vi "ParseStateMsg.vi"(0 "StateMsg":refnum<class "JSON Object.lvclass">, 11 "error in":errorcluster) -> (4 "StateMsg":T1, 15 "error out":errorcluster)   [LabVIEW 2017]
uses:
  <vilib>/NI/JSON Support for LabVIEW/JSON Data Classes/JSON Object/JSON Object.lvclass
  StateMsg.ctl
  <vilib>/NI/JSON Support for LabVIEW/JSON Data Classes/JSON Object/Get Value (Object).vi
  <vilib>/NI/JSON Support for LabVIEW/JSON Data Classes/JSON Object/Get Value (String Value).vi
  <vilib>/NI/JSON Support for LabVIEW/JSON Data Classes/JSON Object/Get Value (Boolean Value).vi
  <vilib>/NI/JSON Support for LabVIEW/JSON Data Classes/JSON Object/Get Value (Numeric Value).vi
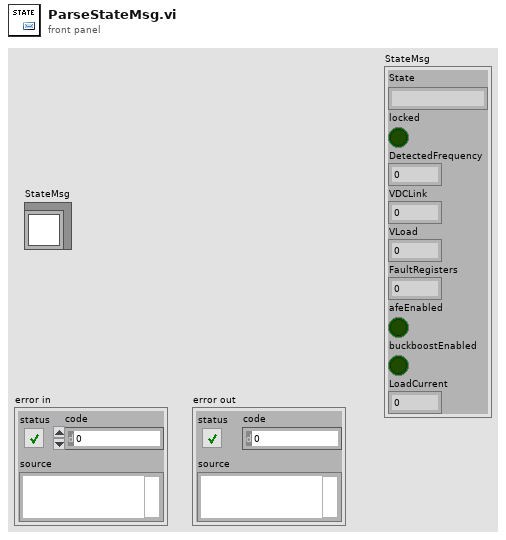
[diagram p1: front panel]
types:
  T1 = typedef "StateMsg.ctl" = cluster{"State":string, "locked":bool, "DetectedFrequency":dbl, "VDCLink":dbl, "VLoad":dbl, "FaultRegisters":u64, "afeEnabled":bool, "buckboostEnabled":bool, "LoadCurrent":dbl}
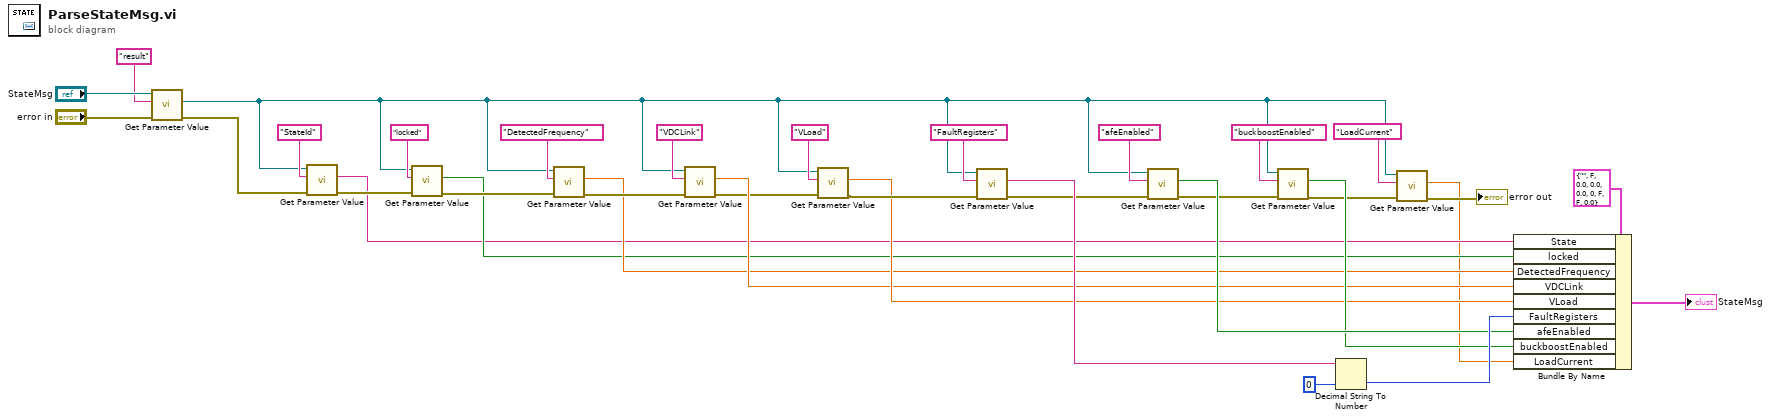
[diagram p0: block diagram]
diagram:
  n1 = call-poly <vilib>:"Get Parameter Value.vi"("error in (no error)"="error in", "key"="result", "JSON Object in"="StateMsg") -> ("error out"=w18:errorcluster, "value"=w5:refnum<class "JSON Object.lvclass">)  [unwired: 7 in]
  n2 = call-poly <vilib>:"Get Parameter Value.vi"("error in (no error)"=w18, "key"="StateId", "JSON Object in"=w5) -> ("error out"=w29:errorcluster, "value"=w6:string)  [unwired: 7 in]
  n3 = call-poly <vilib>:"Get Parameter Value.vi"("error in (no error)"=w29, "key"="locked", "JSON Object in"=w5) -> ("error out"=w28:errorcluster, "value"=w7:bool)  [unwired: 7 in]
  n4 = call-poly <vilib>:"Get Parameter Value.vi"("error in (no error)"=w28, "key"="DetectedFrequency", "JSON Object in"=w5) -> ("error out"=w27:errorcluster, "value"=w8:dbl)  [unwired: 7 in]
  n5 = call-poly <vilib>:"Get Parameter Value.vi"("error in (no error)"=w27, "key"="VDCLink", "JSON Object in"=w5) -> ("error out"=w9:errorcluster, "value"=w10:dbl)  [unwired: 7 in]
  n6 = call-poly <vilib>:"Get Parameter Value.vi"("error in (no error)"=w9, "key"="VLoad", "JSON Object in"=w5) -> ("error out"=w12:errorcluster, "value"=w11:dbl)  [unwired: 7 in]
  n7 = call-poly <vilib>:"Get Parameter Value.vi"("error in (no error)"=w12, "key"="FaultRegisters", "JSON Object in"=w5) -> ("error out"=w13:errorcluster, "value"=w14:string)  [unwired: 7 in]
  n8 = call-poly <vilib>:"Get Parameter Value.vi"("error in (no error)"=w13, "key"="afeEnabled", "JSON Object in"=w5) -> ("error out"=w15:errorcluster, "value"=w17:bool)  [unwired: 7 in]
  n9 = call-poly <vilib>:"Get Parameter Value.vi"("error in (no error)"=w15, "key"="buckboostEnabled", "JSON Object in"=w5) -> ("error out"=w3:errorcluster, "value"=w16:bool)  [unwired: 7 in]
  n10 = Decimal String To Number(string=w14, default (0L)=u64 0) -> (number=w33:u64)  [unwired: 1 in, 1 out]
  n11 = call-poly <vilib>:"Get Parameter Value.vi"("error in (no error)"=w3, "key"="LoadCurrent", "JSON Object in"=w5) -> ("error out"=→"error out":errorcluster, "value"=w1:dbl)  [unwired: 7 in]
  n12 = Bundle By Name(cluster=T1 {"State"="", "locked"=FALSE, "DetectedFrequency"=0.0, "VDCLink"=0.0, "VLoad"=0.0, "FaultRegisters"=0, "afeEnabled"=FALSE, "buckboostEnabled"=FALSE, "LoadCurrent"=0.0} ("StateMsg"), "State"=w6, "locked"=w7, "DetectedFrequency"=w8, "VDCLink"=w10, "VLoad"=w11, "FaultRegisters"=w33, "afeEnabled"=w17, "buckboostEnabled"=w16, "LoadCurrent"=w1) -> (→"StateMsg":T1)
